vi "search_cluster.vi"(10 "change?":bool[](array[boolean]), 11 "Controls[]":refnum<vi>[](array[refnum])) -> (3 "Label.Text":string)   [LabVIEW 2015]
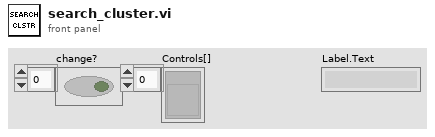
[diagram p1: front panel]
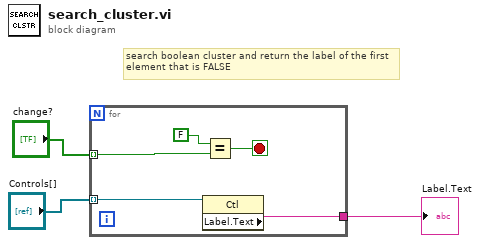
[diagram p0: block diagram]
diagram:
  # "search boolean cluster and return the label of the first element that is FALSE"
  n1 = for {
    tunnel: "Controls[]" -> [w8] mode=indexing
    tunnel: [w7] -> w3
    tunnel: "change?" -> [w5] mode=indexing
    stop <- w6 stop-if-true
    n2 = property class="Ctl"(reference=w8) -> ("Label.Text"=w7:string)  [unwired: 1 in, 2 out]
    n3 = Equal?(x=FALSE, y=w5) -> (x = y?=w6:bool)
  }
  "Label.Text" <- w3
